vi "Create Notifiers.vi"(8 "error in (no error)":errorcluster) -> (0 "error out":errorcluster)   [LabVIEW 2017]
uses:
  Reference Action.ctl
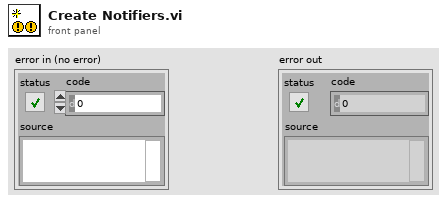
[diagram p1: front panel]
types:
  T1 = typedef "Reference Action.ctl" = enum16{"Set", "Get"}
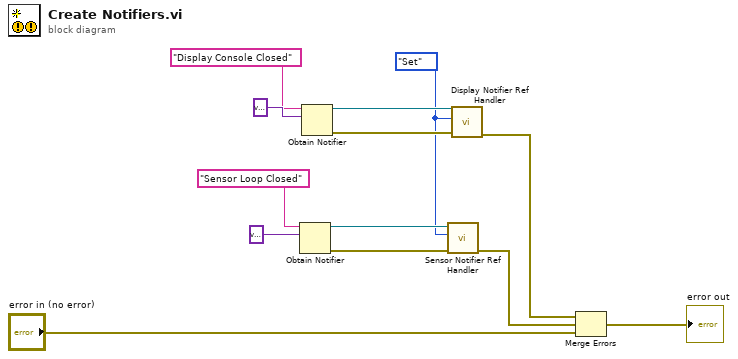
[diagram p0: block diagram]
diagram:
  w4 = Reference_Action."Set" ("Reference Action")
  n1 = Obtain Notifier(name (unnamed)="Sensor Loop Closed", notification data type=variant) -> (notifier out=w5:refnum<notifier>, error out=w6:errorcluster)  [unwired: 2 in, 1 out]
  n2 = Obtain Notifier(name (unnamed)="Display Console Closed", notification data type=variant) -> (notifier out=w8:refnum<notifier>, error out=w7:errorcluster)  [unwired: 2 in, 1 out]
  n3 = call "Sensor Notifier Ref Handler.vi"("Error In"=w6, "Reference Action"=w4, "Notifier Ref In"=w5) -> ("Error Out"=w3:errorcluster)  [unwired: 7 in, 1 out]
  n4 = call "Display Notifier Ref Handler.vi"("Error In"=w7, "Reference Action"=w4, "Notifier Ref In"=w8) -> ("Error Out"=w2:errorcluster)  [unwired: 7 in, 1 out]
  n5 = Merge Errors(w2, w3, "error in (no error)") -> (→"error out":errorcluster)
